vi "System-Integrated Pump.vi"() -> ()   [LabVIEW 2014]
uses:
  <vilib>/LabVIEW Open Source Project/Configuration Manager/Manager/ConfigManager.lvclass
  <vilib>/JKI/JKI SMO/SMO/Typedefs/SMOState --Enum.ctl
  <vilib>/LabVIEW Open Source Project/Configuration Manager/Manager.Text/ConfigManager.Text.lvclass
  <vilib>/JKI/JKI SMO/SMO/SMO.lvclass
  System class/System.lvclass
panel:
  in  "Use ConfigManager.Text":bool
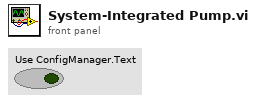
[diagram p1: front panel]
types:
  T1 = typedef "SMO.lvclass/Public Events.ctl" = cluster{"Error":refnum<user-event>, "State":refnum<user-event>, "Reserve State":refnum<user-event>}
  T2 = typedef "SMO.lvclass/SMOState --Enum.ctl" = enum16{"unknown", "Created", "Started", "Stopped"}
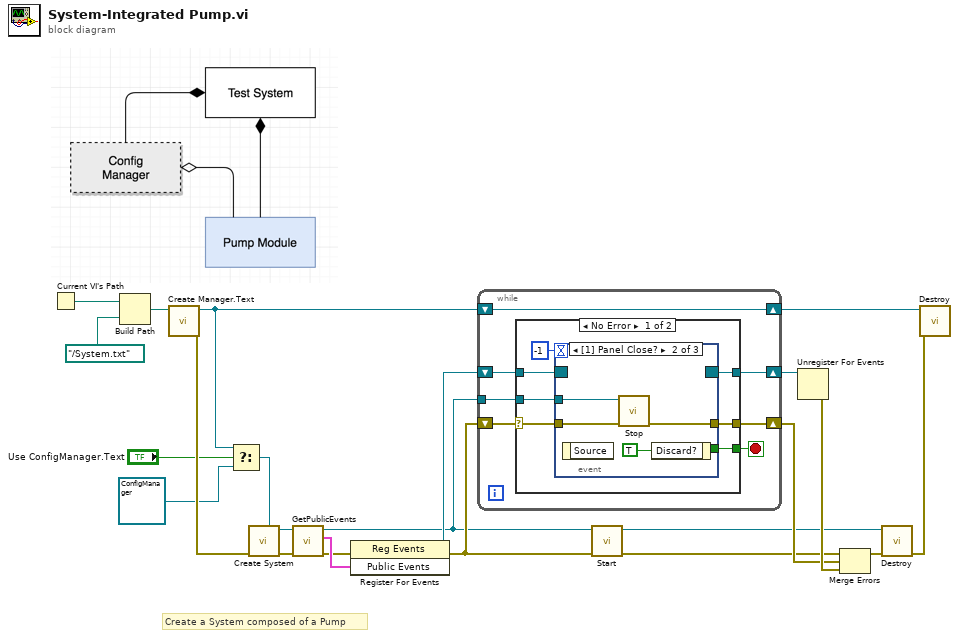
[diagram p0: block diagram]
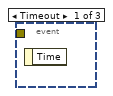
[diagram p2: hidden frame]
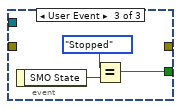
[diagram p3: hidden frame]
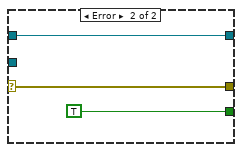
[diagram p4: hidden frame]
diagram:
  # "Create a System composed of a Pump"
  n1 = Current VI's Path() -> (path=w6:path)
  n2 = Build Path(base path=w6, name or relative path=path "../System.txt") -> (appended path=w7:path)
  n3 = call <vilib>:"Create Manager.Text.vi"("filepath"=w7) -> ("error out"=w9:errorcluster, "ConfigManager.Text out"=w3:refnum<class "ConfigManager.Text.lvclass">)  [unwired: 8 in, 1 out]
  n4 = Select(t=w3, s="Use ConfigManager.Text", f=refnum<class "ConfigManager.lvclass"> refnum ("ConfigManager")) -> (s? t:f=w2:refnum<class "ConfigManager.lvclass">)
  n5 = call "Create System.vi"("ConfigManager"=w2, "error in (no error)"=w9) -> ("error out"=w13:errorcluster, "ModuleA out"=w14:refnum<class "System.lvclass">)  [unwired: 7 in, 1 out]
  n6 = call <vilib>:"GetPublicEvents.vi"("error in (no error)"=w13, "SMO"=w14) -> ("error out"=w12:errorcluster, "Public Events"=w23:T1, "SMO out"=w11:refnum<class "System.lvclass">)  [unwired: 7 in]
  n7 = register-events(error in=w12, w23) -> (reference out=w21:refnum<event-registration>, error out=w17:errorcluster)  [unwired: 1 in]
  n8 = while {
    shift-right: [w29] -> w22
    shift-left: w21 -> [w30]
    shift-right: [w26] -> w18
    shift-left: w17 -> [w27]
    tunnel: w11 -> [w25]
    shift-right: [w24] -> w10
    shift-left: w3 -> [w24]
    stop <- w28 stop-if-true
    n9 = case shown="No Error" w27 {
      selector: w27 -> [w32 w45]
      tunnel: w30 -> [w36 w47]
      tunnel: [w35 w47] -> w29
      tunnel: [w34 TRUE] -> w28
      tunnel: [w31 w45] -> w26
      tunnel: w25 -> [w33 _]
      frame No Error {
        n10 = event shown="[1] Panel Close?" {
          selector: w36 -> [_ _ _]
          dyn-events: [_ _ _] -> w35
          timeout: -1 -> [_ _ _]
          tunnel: [_ _ w42] -> w34
          tunnel: w33 -> [_ w41 _]
          tunnel: w32 -> [_ w40 _]
          tunnel: [_ w39 _] -> w31
          event Timeout {
            n11 = event-data() -> ()  [unwired: 1 in, 1 out]
          }
          event Panel Close? {
            n12 = event-data() -> ()  [unwired: 1 in, 1 out]
            n13 = call <vilib>:"Stop.vi"("error in (no error)"=w40, "SMO"=w41) -> ("error out"=w39:errorcluster)  [unwired: 8 in, 1 out]
            n14 = event-data("Discard?"=TRUE) -> ()  [unwired: 1 in, 1 out]
          }
          event User Event {
            n15 = event-data() -> ("SMO State"=w44:T2)  [unwired: 1 in]
            n16 = Equal?(x=SMOState_--Enum."Stopped", y=w44) -> (x = y?=w42:bool)
          }
        }
      }
      frame Error {
      }
    }
  }
  n17 = call <vilib>:"Start.vi"("error in (no error)"=w17, "SMO"=w11) -> ("error out"=w15:errorcluster, "SMO out"=w16:refnum<class "System.lvclass">)  [unwired: 8 in]
  n18 = Unregister For Events(event registration refnum=w22) -> (error out=w19:errorcluster)  [unwired: 1 in]
  n19 = Merge Errors(w15, w18, w19) -> (w20:errorcluster)
  n20 = call <vilib>:"Destroy.vi"("error in (no error)"=w20, "SMO"=w16) -> ("error out"=w8:errorcluster)  [unwired: 9 in]
  n21 = call-dynamic <vilib>:"Destroy.vi"("error in (no error)"=w8, "ConfigManager.Text in"=w10) -> ()  [unwired: 8 in, 2 out]
